vi "Write PXI Mod Instr XML File.vi"() -> ()   [LabVIEW 2009]
doc: "Generates and displays an array of temperature data, and calculates the max, min, and average tempterature. The VI then flattens this data to XML and writes it to a file.\n\n<B>Temp Chart</B> displays the real-time acquisition of data, and <B>Temp Graph</B> displays the data after the VI collects all of the points."
uses:
  <vilib>/Utility/xml.llb/Write to XML File.vi
panel:
  in  "Instr 3 Class Name":string="NI DMM.lvclass"
  in  "Instr 2 Class Name":string="NI Digitizer.lvclass"
  in  "Instr 1 Class Name":string="NI Sig Gen.lvclass"
  out "appended path":path
  in  "XML File Name":string="PXI Mod Instr Config 081226.xml"
  in  "Instr 3 Resource Name":string="NI_DMM_ivi"
  in  "Instr 2 Resource Name":string="NI_Digitizer_ivi"
  in  "Instr 1 Resource Name":string="NI_Sig_Gen_ivi"
  in  "Instr 2 Type":string="Scope"
  in  "Instr 3 Type":string="DMM"
  in  "Instr 1 Type":string="Signal Generator"
  out "XML File Path Out":path
  out "XML Output":string
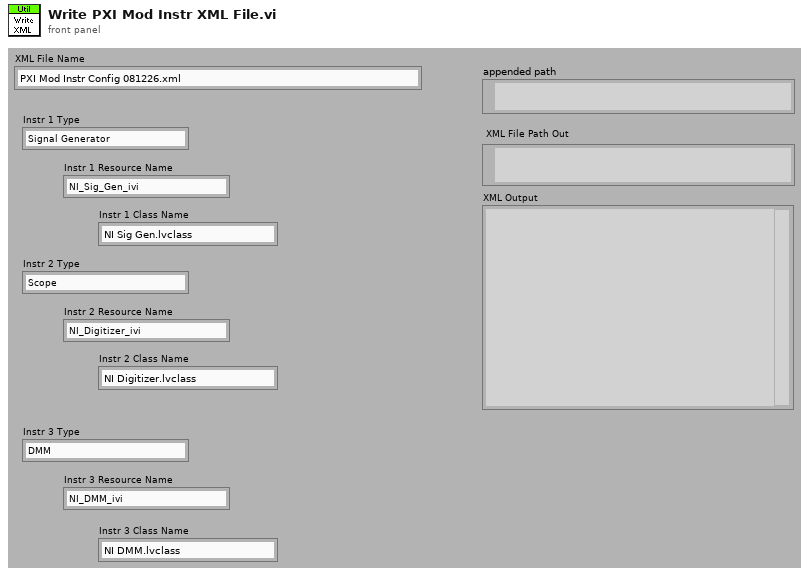
[diagram p1: front panel]
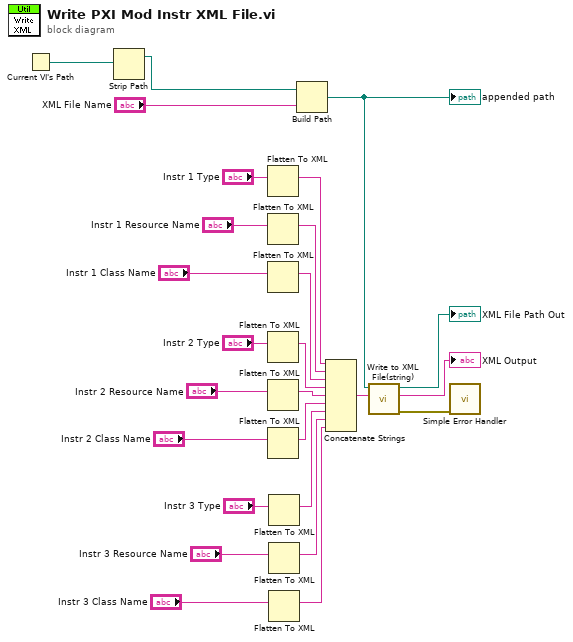
[diagram p0: block diagram]
diagram:
  n1 = Current VI's Path() -> (path=w7:path)
  n2 = Strip Path(path=w7) -> (stripped path=w4:path)  [unwired: 1 out]
  n3 = Flatten To XML(anything="Instr 1 Type") -> (xml string=w26:string)
  n4 = Flatten To XML(anything="Instr 1 Resource Name") -> (xml string=w24:string)
  n5 = Flatten To XML(anything="Instr 1 Class Name") -> (xml string=w23:string)
  n6 = Flatten To XML(anything="Instr 2 Type") -> (xml string=w25:string)
  n7 = Flatten To XML(anything="Instr 2 Resource Name") -> (xml string=w15:string)
  n8 = Flatten To XML(anything="Instr 2 Class Name") -> (xml string=w14:string)
  n9 = Flatten To XML(anything="Instr 3 Type") -> (xml string=w13:string)
  n10 = Flatten To XML(anything="Instr 3 Resource Name") -> (xml string=w12:string)
  n11 = Flatten To XML(anything="Instr 3 Class Name") -> (xml string=w11:string)
  n12 = Build Path(base path=w4, name or relative path="XML File Name") -> (appended path=w5:path)
  "appended path" <- w5
  n13 = Concatenate Strings(w26, w24, w23, w25, w15, w14, w13, w12, w11) -> (w22:string)
  n14 = call-poly <vilib>:"Write to XML File(string).vi"("XML Input"=w22, "XML File Path"=w5) -> ("error out"=w19:errorcluster, "XML String"=→"XML Output":string, "XML File Path(duplicate)"=→"XML File Path Out":path)  [unwired: 3 in, 4 out]
  n15 = call <vilib>:"Simple Error Handler.vi"("error in (no error)"=w19) -> ()  [unwired: 1 in, 8 out]
